vi "Create Error.vi"(7 "source vi name":string, 11 "error":T1=enum."Out of Bounds") -> (1 "new offset":i32, 3 "error out":errorcluster)   [LabVIEW 2027, in "Memory Manager.lvlib" / "Pointer.lvclass"]
uses:
  Pointer.lvclass
  Errors.ctl
  VIs/New Error Cluster (512B).vi
  Constants/Library Name.vi
  Constants/Pointer Class Name.vi
  Static Errors.lvlib
  Memory Manager.lvlib
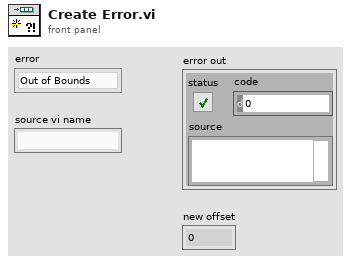
[diagram p1: front panel]
types:
  T1 = typedef "Memory Manager.lvlib/Pointer.lvclass/Errors.ctl" = enum16{"No Error", "Null Pointer", "Out of Bounds", "Buffer Underflow", "Size Mismatch", "Zone"}
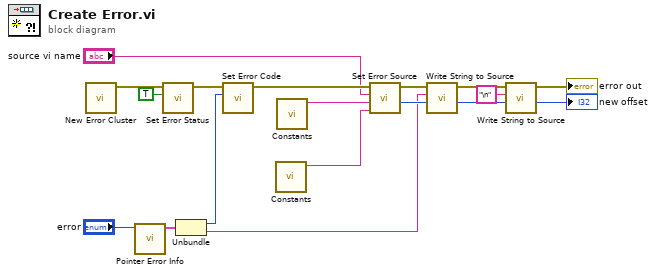
[diagram p0: block diagram]
diagram:
  n1 = call-poly "New Error Cluster.vi"() -> ("error out"=w2:errorcluster)  [unwired: 10 in, 1 out]
  n2 = call "Pointer Error Info.vi"("error"="error") -> ("error info"=w13:cluster{"code":i32, "description":string})  [unwired: 10 in]
  n3 = call "Set Error Status.vi"("status (T)"=TRUE, "error in"=w2) -> ("error out"=w16:errorcluster)  [unwired: 9 in]
  n4 = Unbundle(w13) -> ("code"=w11:i32, "description"=w8:string)
  n5 = call "Set Error Code.vi"("code"=w11, "error in"=w16) -> ("error out"=w17:errorcluster)  [unwired: 9 in]
  n6 = call-poly "Constants.vi"() -> ("pointer class name"=w1:string)  [unwired: 11 in]
  n7 = call-poly "Constants.vi"() -> ("library name"=w18:string)  [unwired: 11 in]
  n8 = call "Set Error Source.vi"("class name (\"\")"=w1, "library name (\"\")"=w18, "vi name"="source vi name", "error in"=w17) -> ("initial offset"=w9:i32, "error out"=w10:errorcluster)  [unwired: 6 in]
  n9 = call "Write String to Source.vi"("offset"=w9, "string"=w8, "error in"=w10) -> ("new offset"=w5:i32, "error out"=w7:errorcluster)  [unwired: 7 in]
  n10 = call "Write String to Source.vi"("offset"=w5, "string"="\n", "error in"=w7) -> ("new offset"=→"new offset":i32, "error out"=→"error out":errorcluster)  [unwired: 7 in]
